vi "Write Multiple Coils.vi"(7 "unit ID":u8, 8 "error in":errorcluster, 9 "coils to write":bool[](array[boolean]), 10 "starting address":u16, 11 "Modbus slave in":refnum<class "Modbus Slave.lvclass">) -> (0 "error out":errorcluster, 3 "Modbus slave out":refnum<class "Modbus Slave.lvclass">)   [LabVIEW 2013, in "Modbus Library - Advance.lvlib" / "Modbus Slave.lvclass"]
doc: "Writes <B>coils to write</B> starting at <B>starting address</B> to the device coils."
uses:
  Modbus Slave.lvclass
  Modbus Slave.lvclass/Modbus Slave.ctl
  Standard Data Model/Standard Data Model.lvclass
  Super Data Model/Super Data Model.lvclass
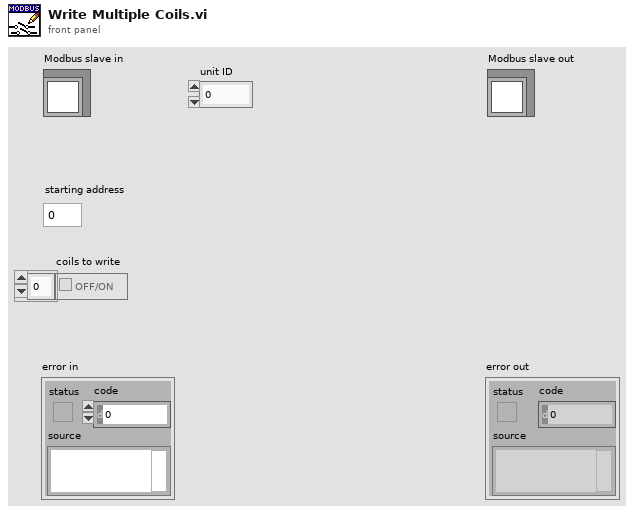
[diagram p1: front panel]
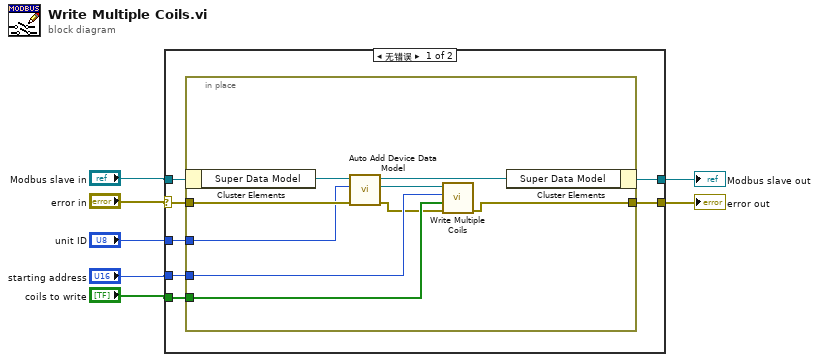
[diagram p0: block diagram]
diagram:
  n1 = case shown="无错误" "error in" {
    selector: "error in" -> [w12 w25]
    tunnel: "coils to write" -> [w14 _]
    tunnel: "starting address" -> [w13 _]
    tunnel: "unit ID" -> [w11 _]
    tunnel: "Modbus slave in" -> [w10 w24]
    tunnel: [w9 w24] -> w7
    tunnel: [w8 w25] -> w6
    frame No Error {
      n2 = in-place {
        in-place-border: w14 -> [w23]
        in-place-border: w13 -> [w22]
        in-place-border: w12 -> [w19]
        in-place-border: [w21] -> w8
        in-place-border: w11 -> [w18]
        n3 = in-place-cluster #1(w10) -> ("Super Data Model"=w20:refnum<class "Super Data Model.lvclass">)
        n4 = call "Auto Add Device Data Model.vi"("error in"=w19, "unit ID"=w18, "Super Data Model in"=w20) -> ("error out"=w16:errorcluster, "device data model"=w15:refnum<class "Standard Data Model.lvclass">, "Super Data Model out"=w17:refnum<class "Super Data Model.lvclass">)  [unwired: 6 in]
        n5 = call-dynamic "Write Multiple Coils.vi"("error in"=w16, "coils"=w23, "starting address"=w22, "device data model in"=w15) -> ("error out"=w21:errorcluster)  [unwired: 6 in, 1 out]
        n6 = in-place-cluster #1("Super Data Model"=w17) -> (w9:refnum<class "Modbus Slave.lvclass">)
      }
    }
    frame Error {
    }
  }
  "error out" <- w6
  "Modbus slave out" <- w7
